vi "FPGA_small2.vi"() -> ()   [LabVIEW 2018]
uses:
  <vilib>/Platform/TimedLoop/XDataNode/timing_clust.ctl
  <vilib>/Platform/TimedLoop/XDataNode/nitl_modes.ctl
  <vilib>/Platform/TimedLoop/XDataNode/wakeup.ctl
  <vilib>/rvi/Emulation/niFpgaGetClockAttributes.vi
  <vilib>/rvi/Emulation/niFpgaSctlEmulationGetInTimedLoop.vi
  <vilib>/rvi/Emulation/niFpgaEmulationReportErrorSimple.vi
  <vilib>/rvi/eio/common/nirviEmuTemplateMethod_errors.vi
  <vilib>/rvi/Emulation/niFpgaCriticalErrorInLSC.vi
  <vilib>/rvi/Emulation/niFpgaProcessEmulError.vi
  <vilib>/eio/EIONode/EIONode.xnode
  <vilib>/platform/TimedLoop/XDataNode/XDataNode.xnode
  <vilib>/Platform/TimedLoop/XDataNode/XDNodeRunTimeDep.lvlib
panel:
  in  "offtrack limit":i16=1500
  out "AI0":u16=1344
  out "dAI":i16=8
  in  "delay ai ms":u32=1
  in  "pwm_val":u32=100
  in  "dt_pwm_us":u32=30 caption="Count(uSec)"
  out "busy":bool
  in  "dt_ctrl_us":u32=1 caption="delay_M_ms"
  in  "set_point":i16
  in  "stop_band":i16=4
  in  "inv":bool=TRUE
  out "gap_pos":i16=-1
  out "backward":bool
  out "position":i16=1241
  out "err cnt":i16
  in  "reset":bool
  out "off_track":bool
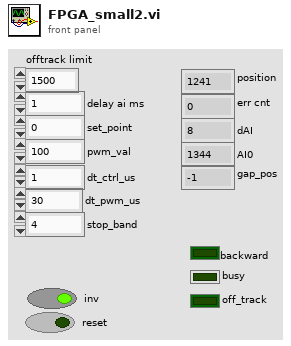
[diagram p1: front panel]
types:
  T1 = typedef "XDNodeRunTimeDep.lvlib/timing_clust.ctl" = cluster{"Expected End [f-1]":u64, "Actual End [f-1]":u64, "Finished Late? [f-1]":bool, "Expected End [i-1]":u64, "Actual End [i-1]":u64, "Finished Late? [i-1]":bool, "Expected Start [i]":u64, "Actual Start [i]":u64, "Expected Start [f]":u64, "Actual Start [f]":u64, "Source Name":string, "Structure Name":string, "Period":i64, "Deadline":i64, "Offset":i64, "Start":i64, "Priority":i32, "Timeout":i32, "Mode":T2, "Wakeup Reason":T3, "Error":errorcluster, "Source Type":string, "Secondary Source Type":string, "Global End Time":u64, "Global Start Time":u64, "Frame Duration":u64, "Iteration Duration":u64, "Assigned CPU":i32, "I/O Scan Engine Mode":u32}
  T2 = typedef "XDNodeRunTimeDep.lvlib/nitl_modes.ctl" = enum32{"No Change", "Process missed periods, maintain original phase", "Discard missed periods, maintain original phase", "Process missed periods, ignore original phase", "Discard missed periods, ignore original phase"}
  T3 = typedef "XDNodeRunTimeDep.lvlib/wakeup.ctl" = enum32{"Normal", "Aborted", "Asynchronous wakeup", "Timing source error", "Timed loop error", "Timeout"}
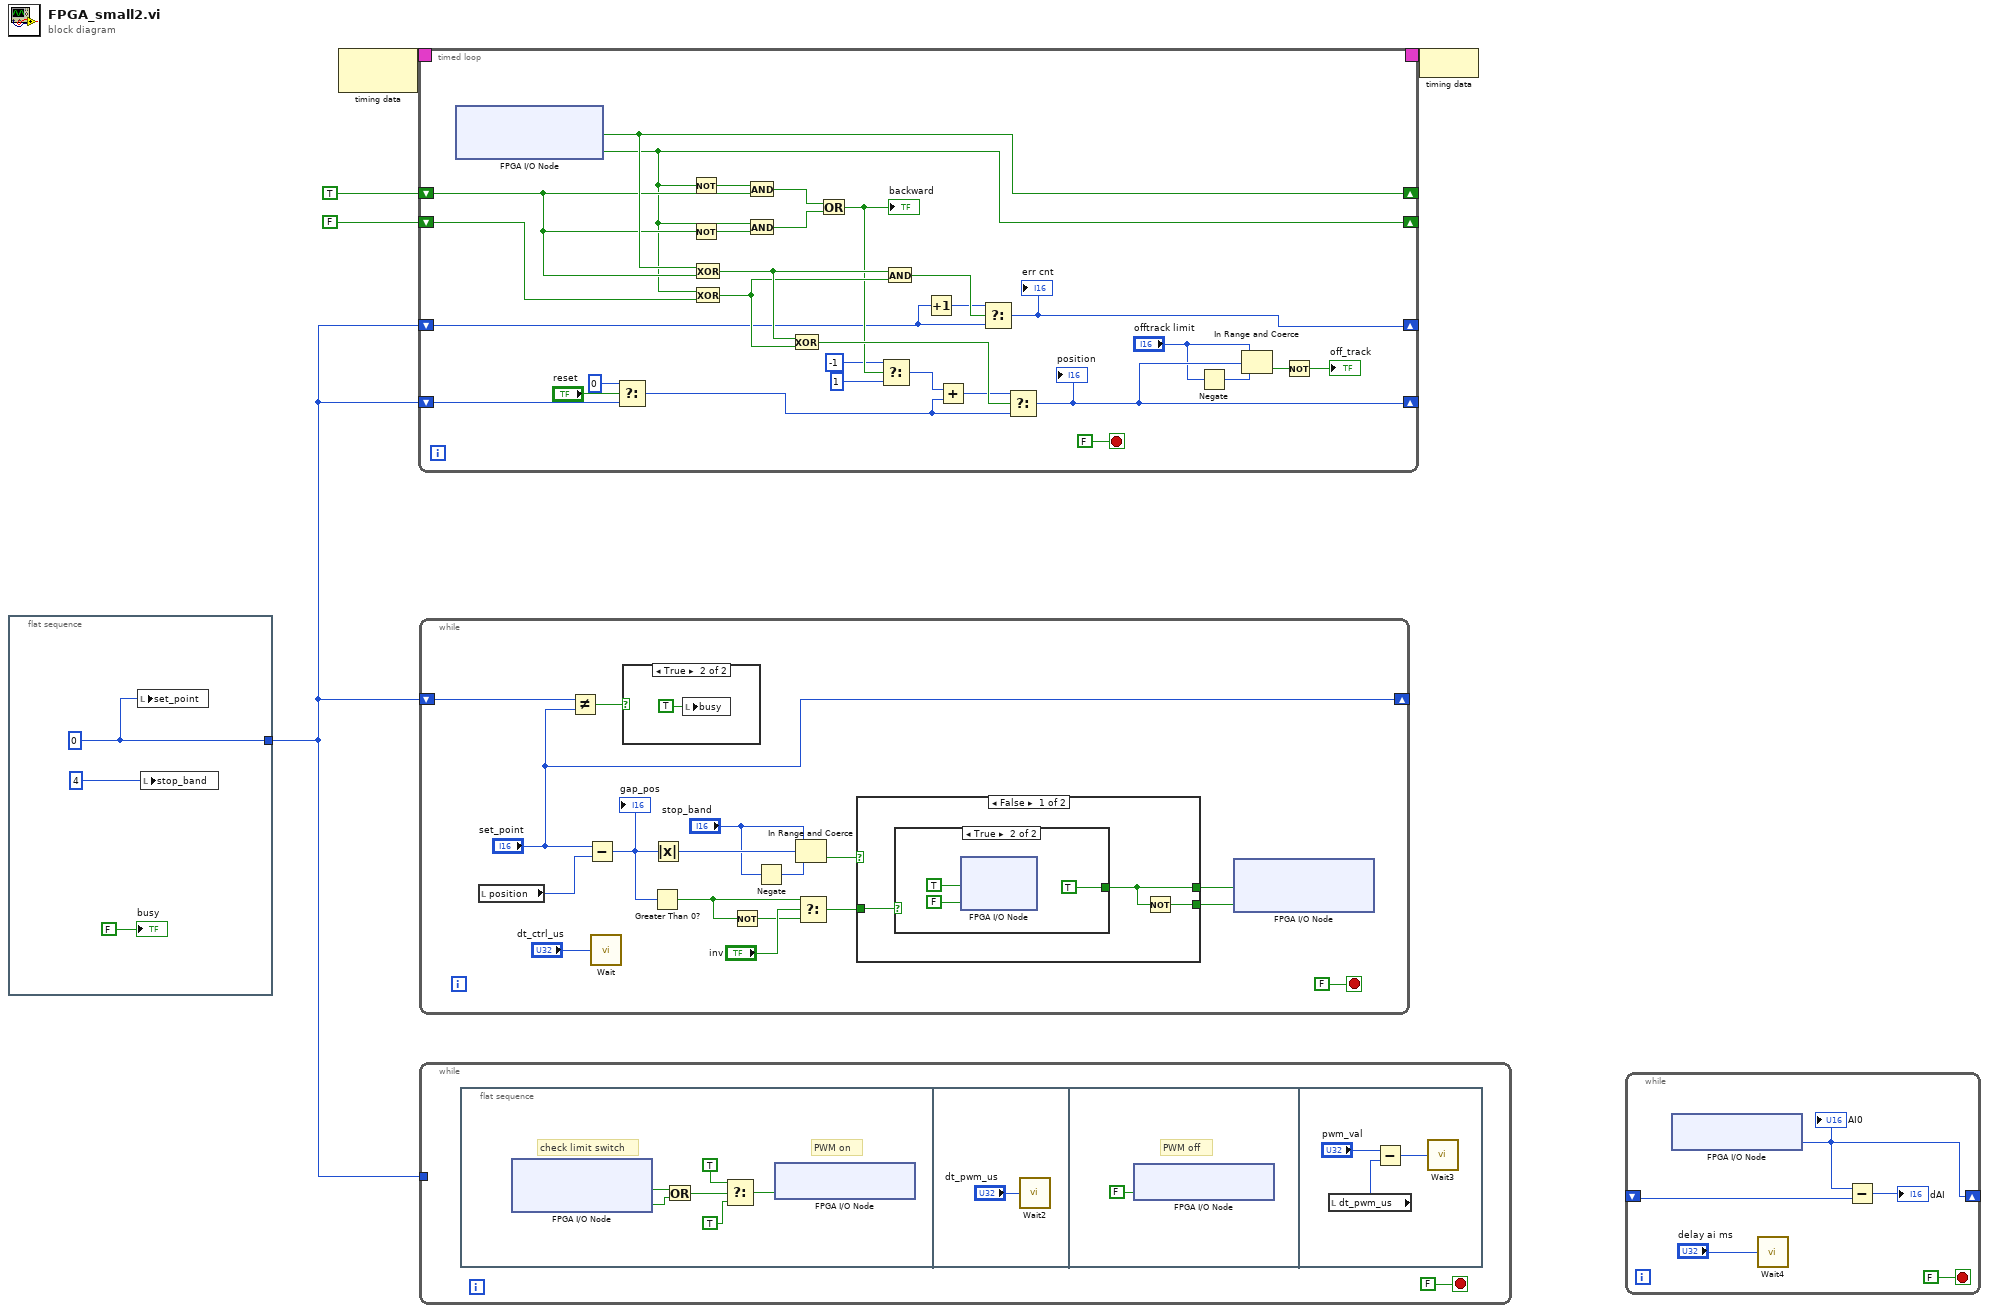
[diagram p0: block diagram]
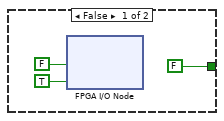
[diagram p3: hidden frame]
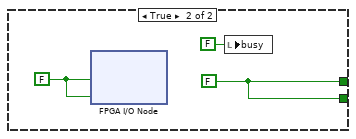
[diagram p4: hidden frame]
diagram:
  n1 = flat-sequence {
    tunnel: [w7] -> w1
    frame #0 {
      w7 = i16 0
      n2 = local write "set_point"(w7) -> ()
      n3 = local write "stop_band"(i16 4 ("dead band")) -> ()
      "busy" <- FALSE ("status")
    }
  }
  n4 = node-c288() -> (w5:T1)  [unwired: 1 in]
  n5 = timed-loop {
    timing: w5 -> [_]
    timing-out: [_] -> w4
    shift-right: [w33] -> _
    shift-left: TRUE ("ConnectorA/DIO11") -> [w32]
    shift-right: [w31] -> _
    shift-left: FALSE ("ConnectorA/DIO12") -> [w30]
    shift-right: [w13] -> _
    shift-left: w1 -> [w16]
    shift-right: [w18] -> _
    shift-left: w1 -> [w19]
    stop <- FALSE stop-if-true
    n6 = xnode "FPGA I/O Node"() -> ("ConnectorA/DIO11"=w33:bool, "ConnectorA/DIO12"=w31:bool)  [unwired: 2 in, 2 out]
    n7 = Select(t=i16 0, s="reset", f=w16) -> (s? t:f=w14:i16)
    n8 = Not(x=w31) -> (.not. x?=w37:bool)
    n9 = Not(x=w32) -> (.not. x?=w36:bool)
    n10 = Exclusive Or(1:w32, 2:w33) -> (0:w29:bool)
    n11 = Exclusive Or(1:w30, 2:w31) -> (0:w28:bool)
    n12 = And(x=w37, y=w32) -> (x .and. y?=w34:bool)
    n13 = And(x=w31, y=w36) -> (x .and. y?=w35:bool)
    n14 = Exclusive Or(1:w28, 2:w29) -> (0:w27:bool)
    n15 = Or(x=w34, y=w35) -> (x .or. y?=w26:bool)
    "backward" <- w26
    n16 = Select(t=i16 -1, s=w26, f=i16 1) -> (s? t:f=w23:i16)
    n17 = And(x=w29, y=w28) -> (x .and. y?=w21:bool)
    n18 = Increment(x=w19) -> (x+1=w20:i16)
    n19 = Add(x=w23, y=w14) -> (x+y=w22:i16)
    n20 = Select(t=w20, s=w21, f=w19) -> (s? t:f=w18:i16)
    "err cnt" <- w18
    n21 = Select(t=w22, s=w27, f=w14) -> (s? t:f=w13:i16)
    "position" <- w13
    n22 = Negate(x="offtrack limit") -> (-x=w10:i16)
    n23 = In Range and Coerce(upper limit="offtrack limit", x=w13, lower limit=w10) -> (In Range?=w12:bool)  [unwired: 1 out]
    n24 = Not(x=w12) -> (.not. x?=→"off_track":bool)
  }
  n25 = while {
    shift-right: ["set_point"] -> _
    shift-left: w1 -> [w42]
    stop <- FALSE stop-if-true
    n26 = local read "position"() -> (w53:i16)
    n27 = Not Equal?(x=w42, y="set_point") -> (x != y?=w41:bool)
    n28 = Subtract(x="set_point", y=w53) -> (x-y=w44:i16)
    "gap_pos" <- w44
    n29 = call "Wait"("Count(uSec)"="dt_ctrl_us") -> ()  [unwired: 1 out]
    n30 = case shown="True" w41 {
      frame False {
      }
      frame True {
        n31 = local write "busy"(TRUE ("busy")) -> ()
      }
    }
    n32 = Greater Than 0?(x=w44) -> (x > 0?=w46:bool)
    n33 = Absolute Value(x=w44) -> (abs(x)=w52:i16)
    n34 = Not(x=w46) -> (.not. x?=w47:bool)
    n35 = Negate(x="stop_band") -> (-x=w51:i16)
    n36 = In Range and Coerce(upper limit="stop_band", x=w52, lower limit=w51) -> (In Range?=w49:bool)  [unwired: 1 out]
    n37 = Select(t=w46, s="inv", f=w47) -> (s? t:f=w45:bool)
    n38 = case shown="False" w49 {
      tunnel: [w61 w70] -> w55
      tunnel: [w60 w70] -> w54
      tunnel: w45 -> [w59 _]
      frame False {
        n39 = case shown="True" w59 {
          tunnel: [FALSE ("dir") TRUE ("dir")] -> w60
          frame False {
            n40 = xnode "FPGA I/O Node"("LED0"=FALSE, "LED1"=TRUE) -> ()  [unwired: 2 in, 2 out]
          }
          frame True {
            n41 = xnode "FPGA I/O Node"("LED0"=TRUE, "LED1"=FALSE) -> ()  [unwired: 2 in, 2 out]
          }
        }
        n42 = Not(x=w60) -> (.not. x?=w61:bool)
      }
      frame True {
        w68 = FALSE ("LED0")
        w70 = FALSE ("dir")
        n43 = xnode "FPGA I/O Node"("LED0"=w68, "LED1"=w68) -> ()  [unwired: 2 in, 2 out]
        n44 = local write "busy"(FALSE ("busy")) -> ()
      }
    }
    n45 = xnode "FPGA I/O Node"("ConnectorA/DIO6"=w54, "ConnectorA/DIO5"=w55) -> ()  [unwired: 2 in, 2 out]
  }
  n46 = while {
    tunnel: w1 -> [_]
    stop <- FALSE stop-if-true
    n47 = flat-sequence {
      frame #0 {
        # "check limit switch"
        # "PWM on"
        n48 = xnode "FPGA I/O Node"() -> ("ConnectorA/DIO0"=w76:bool, "ConnectorA/DIO1"=w77:bool)  [unwired: 2 in, 2 out]
        n49 = Or(x=w76, y=w77) -> (x .or. y?=w75:bool)
        n50 = Select(t=TRUE, s=w75, f=TRUE ("ConnectorA/DIO8")) -> (s? t:f=w74:bool)
        n51 = xnode "FPGA I/O Node"("ConnectorA/DIO8"=w74) -> ()  [unwired: 1 in, 1 out]
      }
      frame #1 {
        n52 = call "Wait2"("Count(uSec)"="dt_pwm_us") -> ()  [unwired: 1 out]
      }
      frame #2 {
        # "PWM off"
        n53 = xnode "FPGA I/O Node"("ConnectorA/DIO8"=FALSE) -> ()  [unwired: 1 in, 1 out]
      }
      frame #3 {
        n54 = local read "dt_pwm_us"() -> (w82:u32)
        n55 = Subtract(x="pwm_val", y=w82) -> (x-y=w80:u32)
        n56 = call "Wait3"("Count(uSec)"=w80) -> ()  [unwired: 1 out]
      }
    }
  }
  n57 = node-c288(w4) -> ()
  n58 = while {
    shift-right: [w84] -> _
    shift-left: _ -> [w85]
    stop <- FALSE stop-if-true
    n59 = xnode "FPGA I/O Node"() -> ("ConnectorA/AI0"=w84:u16)  [unwired: 1 in, 1 out]
    "AI0" <- w84
    n60 = call "Wait4"("Count(mSec)"="delay ai ms") -> ()  [unwired: 1 out]
    n61 = Subtract(x=w84, y=w85) -> (x-y=→"dAI":u16)
  }
